vi "CODMn报警信息转换.vi"(11 "报警簇":T1) -> (1 "code":u64, 2 "CODMN报警信息备注":string, 3 "CODMN报警信息":string)   [LabVIEW 2016, in "斯坦道CODMn.lvlib"]
uses:
  Alarm interface/Alarm interface.lvlib
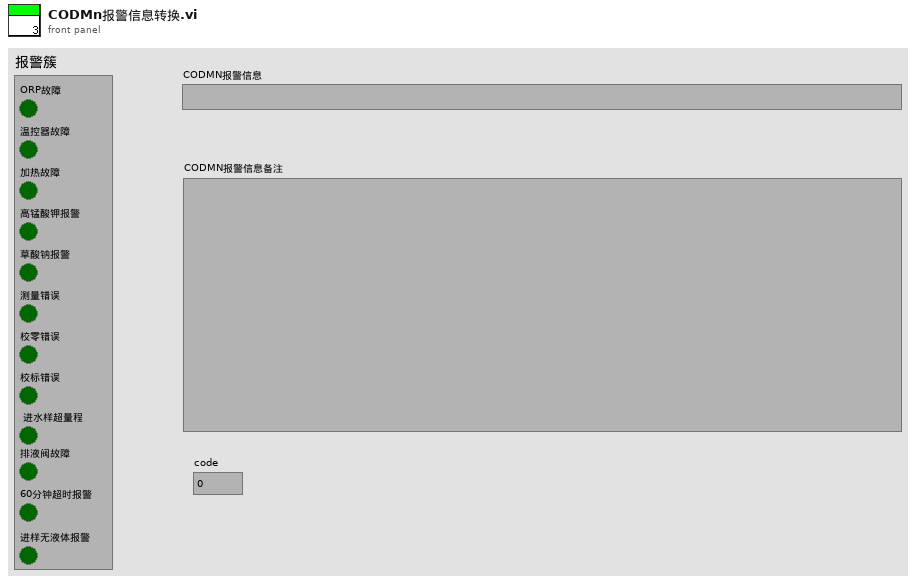
[diagram p1: front panel]
types:
  T1 = cluster{"ORP故障":bool, "温控器故障":bool, "加热故障":bool, "高锰酸钾报警":bool, "草酸钠报警":bool, "测量错误":bool, "校零错误":bool, "校标错误":bool, " 进水样超量程":bool, "排液阀故障":bool, "60分钟超时报警":bool, "进样无液体报警":bool}
  T2 = enum16{"营养盐", "V2CODMn", "新CODMn", "动力环境", "质控单元", "采配水", "其他"}
  T3 = cluster{"modid":i32, "sysid":i32, "content":string, "故障详情":string}
  T4 = cluster{"module name":string, "moduleid":i32, "sysid":i32, "content":string, "analysis":string}
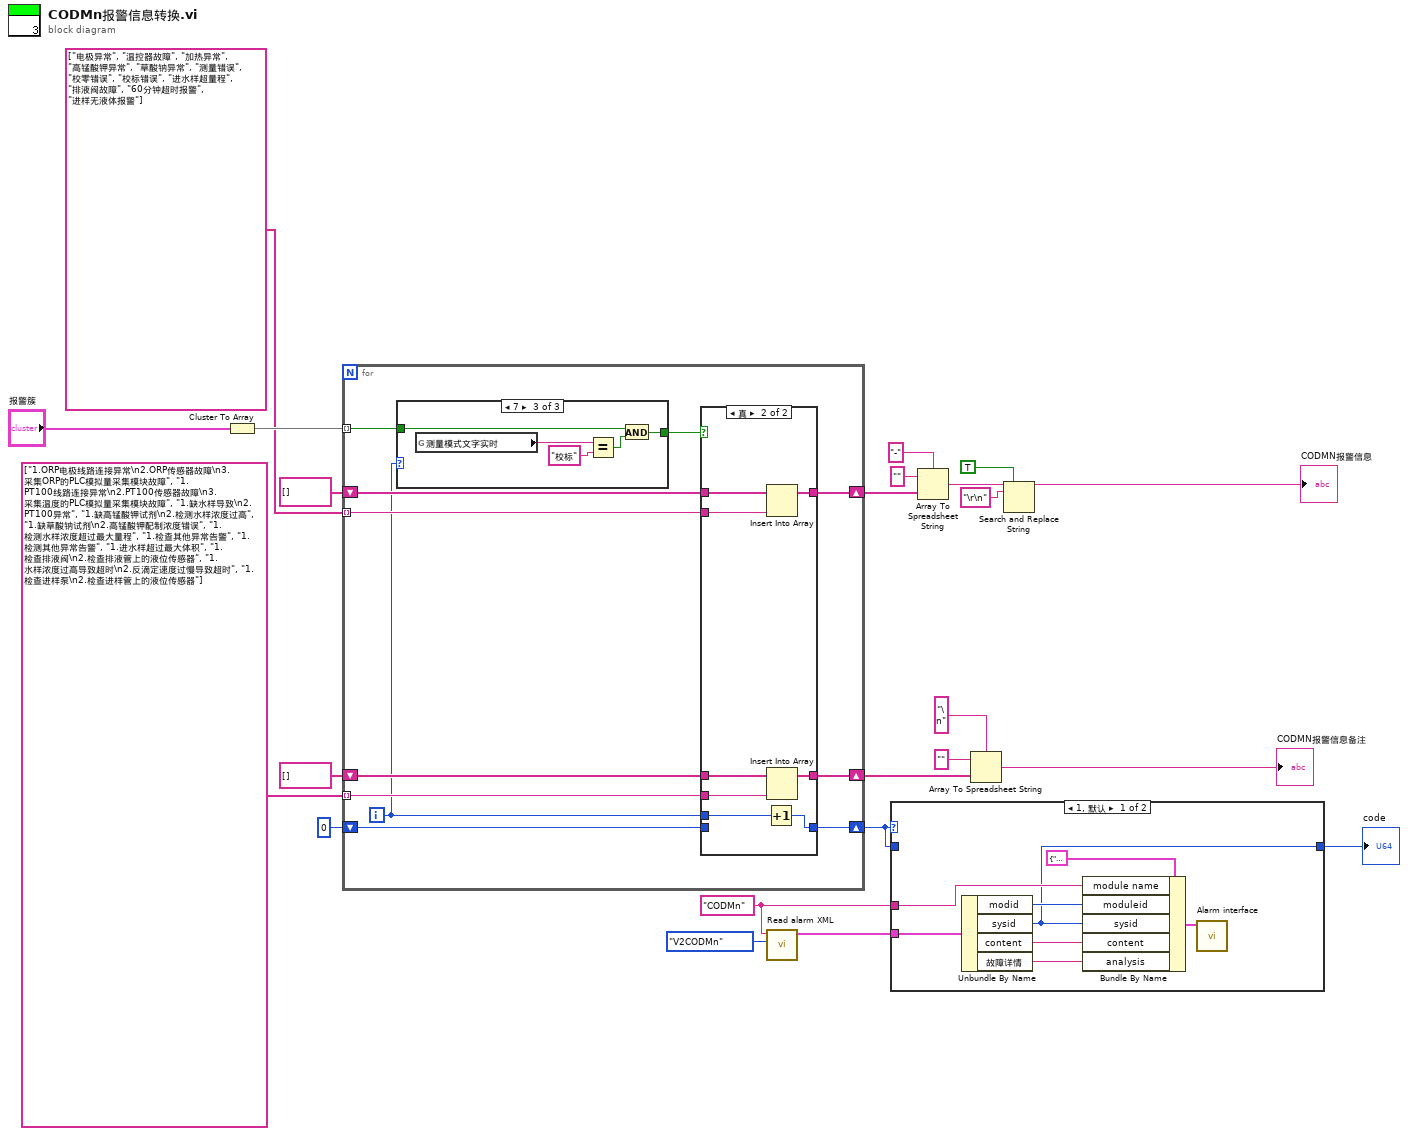
[diagram p0: block diagram]
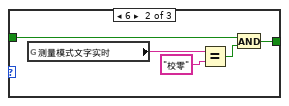
[diagram p4: hidden frame]
diagram:
  w4 = "CODMn" ("模块名称")
  n1 = Cluster To Array(cluster="报警簇") -> (array=w16:bool[])
  n2 = for {
    tunnel: w16 -> [w34] mode=indexing
    shift-right: [w30] -> w11
    shift-left: string[] [] -> [w32]
    tunnel: string[] ["电极异常", "温控器故障", "加热异常", "高锰酸钾异常", "草酸钠异常", "测量错误", "校零错误", "校标错误", "进水样超量程", "排液阀故障", "60分钟超时报警", "进样无液体报警"] -> [w31] mode=indexing
    shift-right: [w27] -> w8
    shift-left: string[] [] -> [w29]
    tunnel: string[] ["1.ORP电极线路连接异常\n2.ORP传感器故障\n3.采集ORP的PLC模拟量采集模块故障", "1.PT100线路连接异常\n2.PT100传感器故障\n3.采集温度的PLC模拟量采集模块故障", "1.缺水样导致\n2.PT100异常", "1.缺高锰酸钾试剂\n2.检测水样浓度过高", "1.缺草酸钠试剂\n2.高锰酸钾配制浓度错误", "1.检测水样浓度超过最大量程", "1.检查其他异常告警", "1.检测其他异常告警", "1.进水样超过最大体积", "1.检查排液阀\n2.检查排液管上的液位传感器", "1.水样浓度过高导致超时\n2.反滴定速度过慢导致超时", "1.检查进样泵\n2.检查进样管上的液位传感器"] -> [w28] mode=indexing
    shift-right: [w25] -> w1
    shift-left: 0 -> [w24]
    i -> [w26]
    n3 = case shown="7" w26 {
      tunnel: w34 -> [w35 w37 w42]
      tunnel: [w35 w36 w41] -> w33
      frame 0, Default {
      }
      frame 6 {
        n4 = global read "COD测量模式全局.vi" "测量模式文字实时"() -> (w39:string)
        n5 = Equal?(x=w39, y="校零" ("测量模式")) -> (x = y?=w38:bool)
        n6 = And(x=w37, y=w38) -> (x .and. y?=w36:bool)
      }
      frame 7 {
        n7 = global read "COD测量模式全局.vi" "测量模式文字实时"() -> (w44:string)
        n8 = Equal?(x=w44, y="校标" ("测量模式")) -> (x = y?=w43:bool)
        n9 = And(x=w42, y=w43) -> (x .and. y?=w41:bool)
      }
    }
    n10 = case shown="真" w33 {
      tunnel: w32 -> [w48 w56]
      tunnel: w31 -> [_ w55]
      tunnel: [w48 w54] -> w30
      tunnel: w29 -> [w47 w53]
      tunnel: w28 -> [_ w52]
      tunnel: [w47 w51] -> w27
      tunnel: w26 -> [_ w50]
      tunnel: [w46 w49] -> w25
      tunnel: w24 -> [w46 _]
      frame False {
      }
      frame True {
        n11 = Increment(x=w50) -> (x+1=w49:i32)
        n12 = Insert Into Array(array=w56, new element=w55) -> (w54:string[])  [unwired: 1 in]
        n13 = Insert Into Array(array=w53, new element=w52) -> (w51:string[])  [unwired: 1 in]
      }
    }
  }
  n14 = call "Read alarm XML.vi"("模块常量"=T2."V2CODMn", "模块名称"=w4) -> ("报警"=w5:T3)  [unwired: 9 in]
  n15 = case shown="1, 默认" w1 {
    tunnel: w5 -> [w61 _]
    tunnel: w4 -> [w63 _]
    tunnel: [w59 w65] -> w2
    tunnel: w1 -> [_ w65]
    frame 1, Default {
      n16 = Unbundle By Name(w61) -> ("modid"=w60:i32, "sysid"=w59:i32, "content"=w58:string, "故障详情"=w57:string)
      n17 = Bundle By Name(cluster=T4 {"module name"="", "moduleid"=0, "sysid"=0, "content"="", "analysis"=""} ("簇"), "module name"=w63, "moduleid"=w60, "sysid"=w59, "content"=w58, "analysis"=w57) -> (w62:T4)
      n18 = call "Alarm interface.vi"("簇"=w62) -> ()  [unwired: 10 in, 1 out]
    }
    frame -1 {
    }
  }
  "code" <- w2
  n19 = Array To Spreadsheet String(delimiter (Tab)="-" ("分隔符(Tab)"), array=w11, 3:"" ("格式字符串")) -> (spreadsheet string=w19:string)
  n20 = Array To Spreadsheet String(delimiter (Tab)="\n" ("分隔符(Tab)"), array=w8, 3:"" ("格式字符串")) -> (spreadsheet string=→"CODMN报警信息备注":string)
  n21 = Search and Replace String(replace all?=TRUE ("替换全部？(F)"), input string=w19, search string="\r\n" ("搜索字符串")) -> (result string=→"CODMN报警信息":string)  [unwired: 5 in, 3 out]
